vi "AlGaInPAs_Layer.vi"(2 "Debug Mode":bool, 3 "Elapsed Time (s)":dbl, 4 "State":enum16{"Edit", "Start", "Run", "End", "Idle"}(ring), 5 "Argument List In":string[](array[string])) -> (0 "Status Out":string, 1 "Argument List Out":string[](array[string]))   [LabVIEW 2011]
panel:
  out "Al?":bool
  out "In?":bool
  out "Ga?":bool
  out "AsH3?":bool
  out "PH3?":bool
  in  "AsH3 Flow":dbl
  in  "AsH3 run":bool
  in  "Al_run":bool
  in  "Al Flow":dbl
  in  "PH3 run":bool
  in  "In run":bool
  in  "Ga run":bool
  in  "PH3 Flow":dbl
  in  "In Flow":dbl
  in  "Ga Flow":dbl
  in  "Cancel":bool
  in  "OK":bool
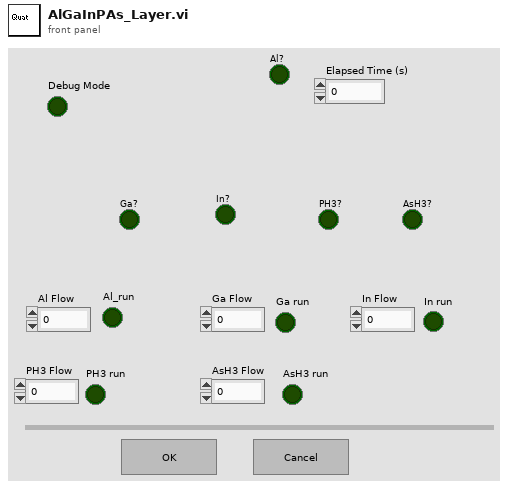
[diagram p1: front panel]
types:
  T1 = enum16{"Discrete", "Continuous", "Instantaneous"}
  T2 = enum32{"Invalid", "Default", "Floating", "Floating/Auto-Hide", "Modal"}
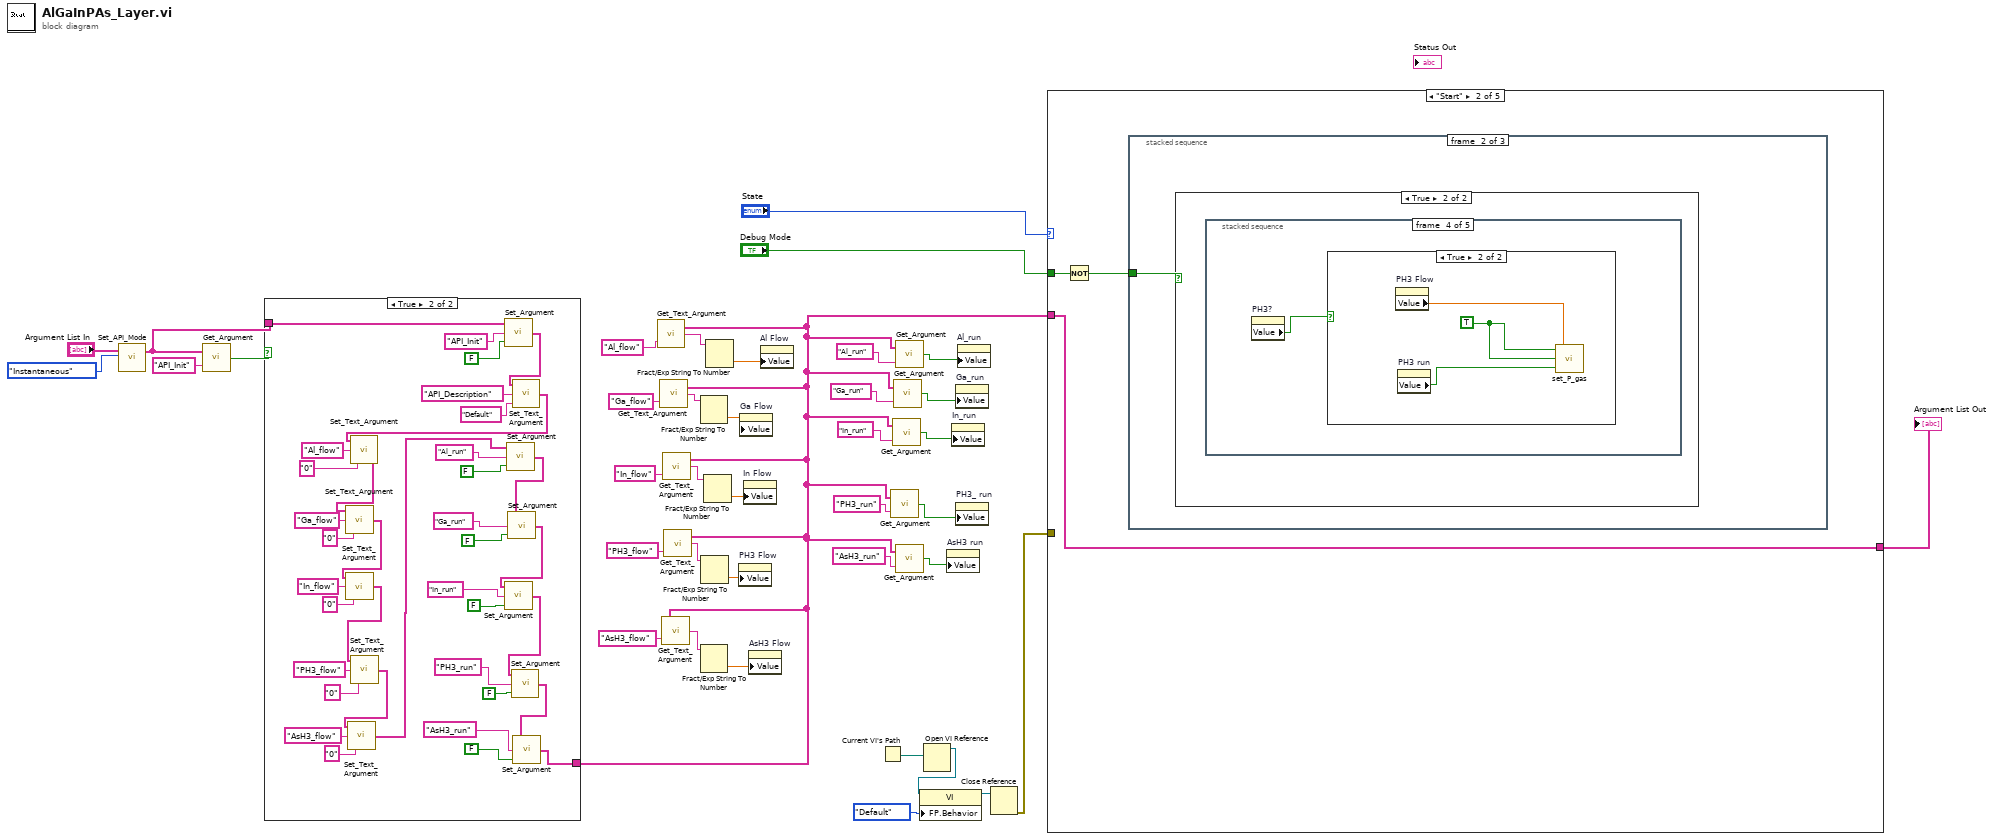
[diagram p0: block diagram]
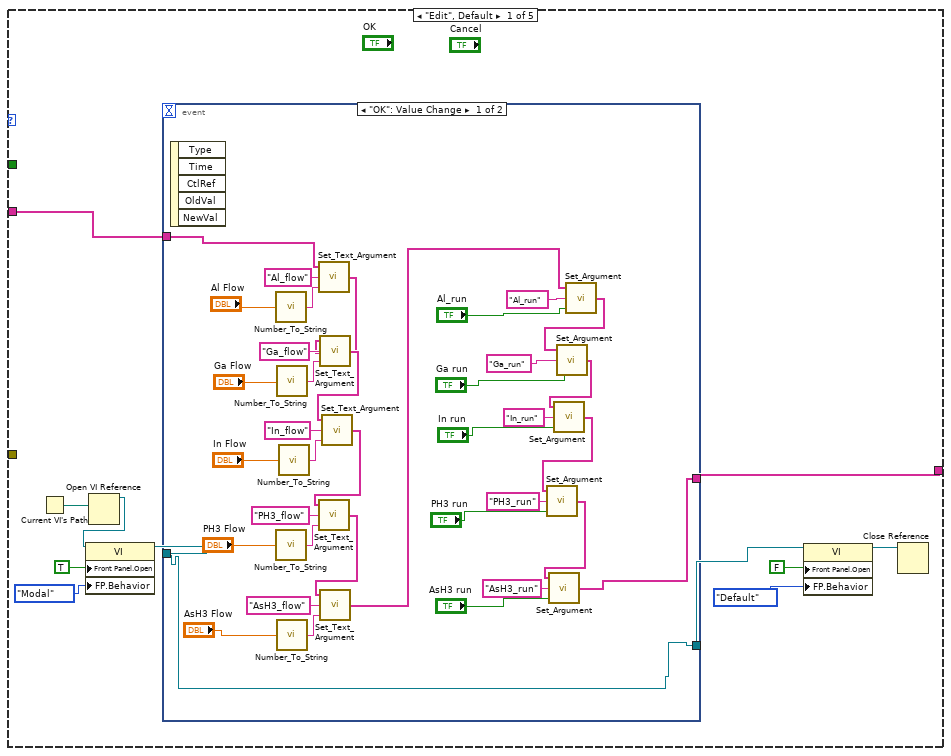
[diagram p3: hidden frame]
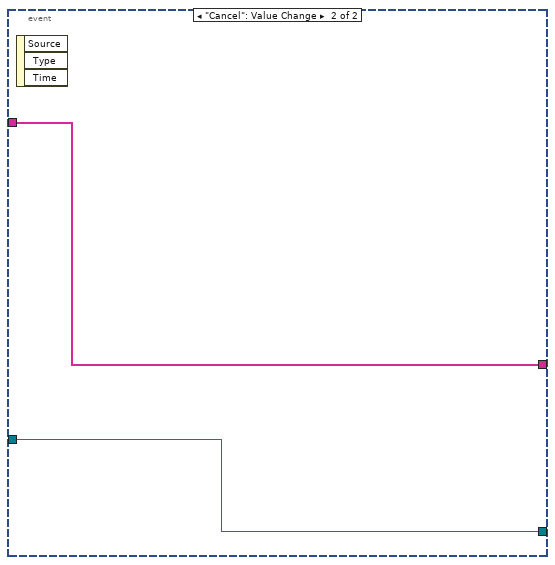
[diagram p4: hidden frame]
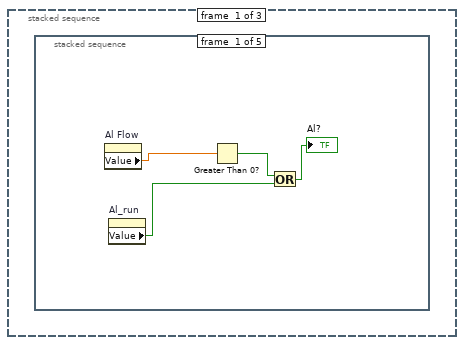
[diagram p5: hidden frame]
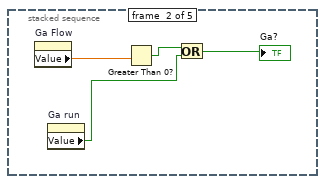
[diagram p6: hidden frame]
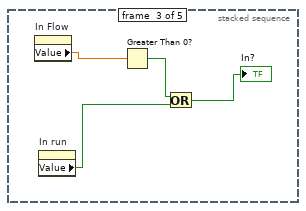
[diagram p7: hidden frame]
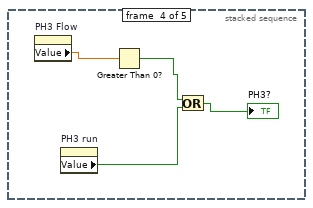
[diagram p8: hidden frame]
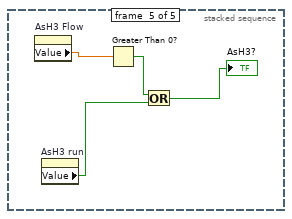
[diagram p9: hidden frame]
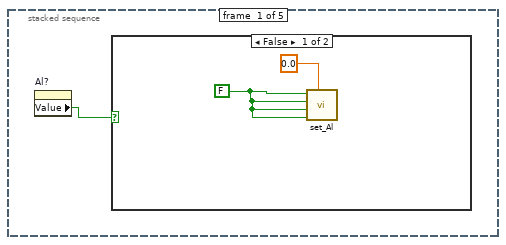
[diagram p11: hidden frame]
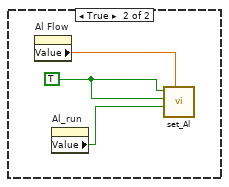
[diagram p12: hidden frame]
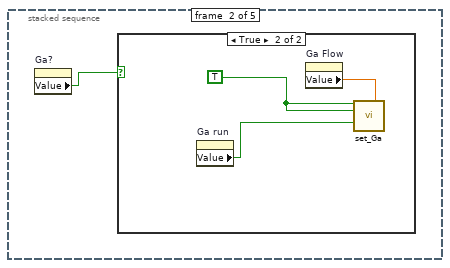
[diagram p13: hidden frame]
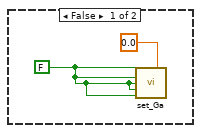
[diagram p14: hidden frame]
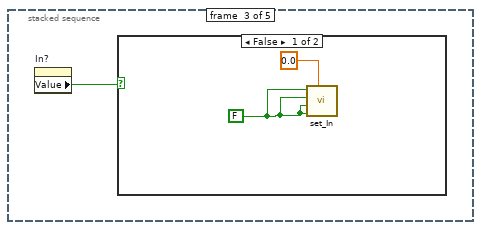
[diagram p15: hidden frame]
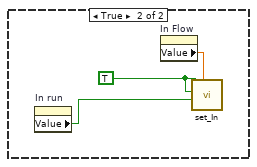
[diagram p16: hidden frame]
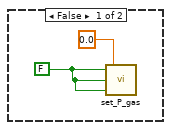
[diagram p17: hidden frame]
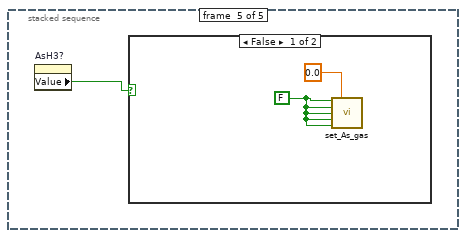
[diagram p18: hidden frame]
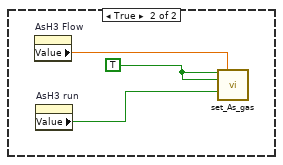
[diagram p19: hidden frame]
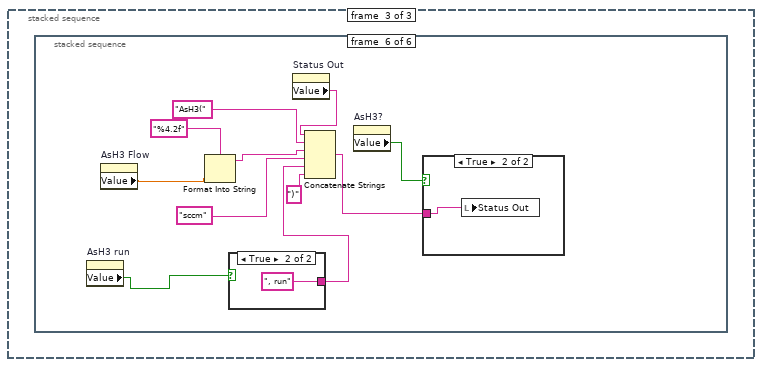
[diagram p20: hidden frame]
diagram:
  n1 = call "Set_API_Mode.vi"("API Mode"=T1."Instantaneous", "Argument List In"="Argument List In") -> ("Argument List Out"=w26:string[])  [unwired: 3 in]
  n2 = call "Get_Argument.vi"("Argument"="API_Init", "Argument List"=w26) -> ("Enabled"=w27:bool)
  n3 = case shown="True" w27 {
    tunnel: w26 -> [w40 w77]
    tunnel: [w40 w53] -> w1
    frame False {
    }
    frame True {
      n4 = call "Set_Argument.vi"("Enable"=FALSE, "Argument"="API_Init", "Argument List In"=w77) -> ("Argument List Out"=w74:string[])
      n5 = call "Set_Text_Argument.vi"("Text"="Default", "Argument"="API_Description", "Argument List In"=w74) -> ("Argument List Out"=w45:string[])
      n6 = call "Set_Text_Argument.vi"("Text"="0", "Argument"="Al_flow", "Argument List In"=w45) -> ("Argument List Out"=w44:string[])
      n7 = call "Set_Text_Argument.vi"("Text"="0", "Argument"="Ga_flow", "Argument List In"=w44) -> ("Argument List Out"=w67:string[])
      n8 = call "Set_Text_Argument.vi"("Text"="0", "Argument"="In_flow", "Argument List In"=w67) -> ("Argument List Out"=w43:string[])
      n9 = call "Set_Text_Argument.vi"("Text"="0", "Argument"="PH3_flow", "Argument List In"=w43) -> ("Argument List Out"=w55:string[])
      n10 = call "Set_Text_Argument.vi"("Text"="0", "Argument"="AsH3_flow", "Argument List In"=w55) -> ("Argument List Out"=w42:string[])
      n11 = call "Set_Argument.vi"("Enable"=FALSE, "Argument"="Al_run", "Argument List In"=w42) -> ("Argument List Out"=w48:string[])
      n12 = call "Set_Argument.vi"("Enable"=FALSE, "Argument"="Ga_run", "Argument List In"=w48) -> ("Argument List Out"=w58:string[])
      n13 = call "Set_Argument.vi"("Enable"=FALSE, "Argument"="In_run", "Argument List In"=w58) -> ("Argument List Out"=w41:string[])
      n14 = call "Set_Argument.vi"("Enable"=FALSE, "Argument"="PH3_run", "Argument List In"=w41) -> ("Argument List Out"=w51:string[])
      n15 = call "Set_Argument.vi"("Enable"=FALSE, "Argument"="AsH3_run", "Argument List In"=w51) -> ("Argument List Out"=w53:string[])
    }
  }
  n16 = call "Get_Text_Argument.vi"("Argument"="Al_flow", "Argument List"=w1) -> ("Text"=w6:string)
  n17 = call "Get_Text_Argument.vi"("Argument"="Ga_flow", "Argument List"=w1) -> ("Text"=w22:string)
  n18 = call "Get_Text_Argument.vi"("Argument"="AsH3_flow", "Argument List"=w1) -> ("Text"=w18:string)
  n19 = call "Get_Text_Argument.vi"("Argument"="In_flow", "Argument List"=w1) -> ("Text"=w20:string)
  n20 = call "Get_Text_Argument.vi"("Argument"="PH3_flow", "Argument List"=w1) -> ("Text"=w17:string)
  n21 = Fract/Exp String To Number(string=w22) -> (number=w21:dbl)  [unwired: 4 out]
  n22 = Fract/Exp String To Number(string=w18) -> (number=w2:dbl)  [unwired: 4 out]
  n23 = Fract/Exp String To Number(string=w17) -> (number=w16:dbl)  [unwired: 4 out]
  n24 = Fract/Exp String To Number(string=w20) -> (number=w19:dbl)  [unwired: 4 out]
  n25 = Fract/Exp String To Number(string=w6) -> (number=w3:dbl)  [unwired: 4 out]
  n26 = property on="PH3 Flow" class="DigNum (strict)"("Value"=w16) -> ()  [unwired: 2 in, 2 out]
  n27 = property on="Ga Flow" class="DigNum (strict)"("Value"=w21) -> ()  [unwired: 2 in, 2 out]
  n28 = property on="In Flow" class="DigNum (strict)"("Value"=w19) -> ()  [unwired: 2 in, 2 out]
  n29 = property on="AsH3 Flow" class="DigNum (strict)"("Value"=w2) -> ()  [unwired: 2 in, 2 out]
  n30 = property on="Al Flow" class="DigNum (strict)"("Value"=w3) -> ()  [unwired: 2 in, 2 out]
  n31 = Current VI's Path() -> (path=w35:path)
  n32 = call "Get_Argument.vi"("Argument"="PH3_run", "Argument List"=w1) -> ("Enabled"=w12:bool)
  n33 = call "Get_Argument.vi"("Argument"="In_run", "Argument List"=w1) -> ("Enabled"=w13:bool)
  n34 = call "Get_Argument.vi"("Argument"="Ga_run", "Argument List"=w1) -> ("Enabled"=w14:bool)
  n35 = call "Get_Argument.vi"("Argument"="Al_run", "Argument List"=w1) -> ("Enabled"=w5:bool)
  n36 = call "Get_Argument.vi"("Argument"="AsH3_run", "Argument List"=w1) -> ("Enabled"=w4:bool)
  n37 = Open VI Reference(vi path=w35) -> (vi reference=w34:refnum<vi>)  [unwired: 1 in, 5 out]
  n38 = property class="VI"(reference=w34, "FP.Behavior"=T2."Default" ("Front Panel Window:Behavior")) -> (reference out=w32:refnum<vi>)  [unwired: 1 in, 1 out]
  n39 = property on="AsH3 run" class="Bool (strict)"("Value"=w4) -> ()  [unwired: 2 in, 2 out]
  n40 = property on="In_run" class="Bool (strict)"("Value"=w13) -> ()  [unwired: 2 in, 2 out]
  n41 = property on="Ga_run" class="Bool (strict)"("Value"=w14) -> ()  [unwired: 2 in, 2 out]
  n42 = property on="PH3_ run" class="Bool (strict)"("Value"=w12) -> ()  [unwired: 2 in, 2 out]
  n43 = property on="Al_run" class="Bool (strict)"("Value"=w5) -> ()  [unwired: 2 in, 2 out]
  n44 = Close Reference(reference=w32) -> (error out=w31:errorcluster)  [unwired: 1 in]
  n45 = case shown="\"Start\"" "State" {
    tunnel: [w88 w130 w252 w253 w254] -> w38
    tunnel: w1 -> [w87 w130 w252 w253 w254]
    tunnel: "Debug Mode" -> [_ w129 _ _ _]
    tunnel: w31 -> [_ _ _ _ _]
    frame "Edit", Default {
      n46 = Current VI's Path() -> (path=w82:path)
      n47 = Open VI Reference(vi path=w82) -> (vi reference=w81:refnum<vi>)  [unwired: 1 in, 5 out]
      n48 = property class="VI"(reference=w81, "Front Panel.Open"=TRUE ("Front Panel Window:Open"), "FP.Behavior"=T2."Modal" ("Front Panel Window:Behavior")) -> (reference out=w85:refnum<vi>)  [unwired: 1 in, 1 out]
      n49 = event shown="[0] \"OK\": Value Change" {
        selector: _ -> [_ _]
        dyn-events: _ -> [_ _]
        timeout: _ -> [_ _]
        tunnel: w87 -> [w98 w126]
        tunnel: [w105 w126] -> w88
        tunnel: [w89 w127] -> w84
        tunnel: w85 -> [w89 w127]
        event "OK": Value Change {
          n50 = event-data() -> ()  [unwired: 6 out]
          n51 = call "Number_To_String.vi"("Number"="Al Flow") -> ("String"=w99:string)
          n52 = call "Number_To_String.vi"("Number"="PH3 Flow") -> ("String"=w117:string)
          n53 = call "Number_To_String.vi"("Number"="Ga Flow") -> ("String"=w124:string)
          n54 = call "Number_To_String.vi"("Number"="AsH3 Flow") -> ("String"=w95:string)
          n55 = call "Number_To_String.vi"("Number"="In Flow") -> ("String"=w121:string)
          n56 = call "Set_Text_Argument.vi"("Text"=w99, "Argument"="Al_flow", "Argument List In"=w98) -> ("Argument List Out"=w97:string[])
          n57 = call "Set_Text_Argument.vi"("Text"=w124, "Argument"="Ga_flow", "Argument List In"=w97) -> ("Argument List Out"=w120:string[])
          n58 = call "Set_Text_Argument.vi"("Text"=w121, "Argument"="In_flow", "Argument List In"=w120) -> ("Argument List Out"=w92:string[])
          n59 = call "Set_Text_Argument.vi"("Text"=w117, "Argument"="PH3_flow", "Argument List In"=w92) -> ("Argument List Out"=w93:string[])
          n60 = call "Set_Text_Argument.vi"("Text"=w95, "Argument"="AsH3_flow", "Argument List In"=w93) -> ("Argument List Out"=w94:string[])
          n61 = call "Set_Argument.vi"("Enable"="Al_run", "Argument"="Al_run", "Argument List In"=w94) -> ("Argument List Out"=w91:string[])
          n62 = call "Set_Argument.vi"("Enable"="Ga run", "Argument"="Ga_run", "Argument List In"=w91) -> ("Argument List Out"=w109:string[])
          n63 = call "Set_Argument.vi"("Enable"="In run", "Argument"="In_run", "Argument List In"=w109) -> ("Argument List Out"=w103:string[])
          n64 = call "Set_Argument.vi"("Enable"="PH3 run", "Argument"="PH3_run", "Argument List In"=w103) -> ("Argument List Out"=w104:string[])
          n65 = call "Set_Argument.vi"("Enable"="AsH3 run", "Argument"="AsH3_run", "Argument List In"=w104) -> ("Argument List Out"=w105:string[])
        }
        event "Cancel": Value Change {
          n66 = event-data() -> ()  [unwired: 4 out]
        }
      }
      n67 = property class="VI"(reference=w84, "Front Panel.Open"=FALSE ("Front Panel Window:Open"), "FP.Behavior"=T2."Default" ("Front Panel Window:Behavior")) -> (reference out=w78:refnum<vi>)  [unwired: 1 in, 1 out]
      n68 = Close Reference(reference=w78) -> ()  [unwired: 1 in, 1 out]
    }
    frame "Start" {
      n69 = Not(x=w129) -> (.not. x?=w128:bool)
      n70 = stacked-sequence {
        tunnel: w128 -> [_ w151 _]
        frame #0 {
          n71 = stacked-sequence {
            frame #0 {
              n72 = property on="Al Flow" class="DigNum (strict)"() -> ("Value"=w131:dbl)  [unwired: 2 in, 2 out]
              n73 = property on="Al_run" class="Bool (strict)"() -> ("Value"=w132:bool)  [unwired: 2 in, 2 out]
              n74 = Greater Than 0?(x=w131) -> (x > 0?=w134:bool)
              n75 = Or(x=w134, y=w132) -> (x .or. y?=→"Al?":bool)
            }
            frame #1 {
              n76 = property on="Ga Flow" class="DigNum (strict)"() -> ("Value"=w138:dbl)  [unwired: 2 in, 2 out]
              n77 = property on="Ga run" class="Bool (strict)"() -> ("Value"=w136:bool)  [unwired: 2 in, 2 out]
              n78 = Greater Than 0?(x=w138) -> (x > 0?=w137:bool)
              n79 = Or(x=w137, y=w136) -> (x .or. y?=→"Ga?":bool)
            }
            frame #2 {
              n80 = property on="In Flow" class="DigNum (strict)"() -> ("Value"=w142:dbl)  [unwired: 2 in, 2 out]
              n81 = property on="In run" class="Bool (strict)"() -> ("Value"=w140:bool)  [unwired: 2 in, 2 out]
              n82 = Greater Than 0?(x=w142) -> (x > 0?=w141:bool)
              n83 = Or(x=w141, y=w140) -> (x .or. y?=→"In?":bool)
            }
            frame #3 {
              n84 = property on="PH3 Flow" class="DigNum (strict)"() -> ("Value"=w146:dbl)  [unwired: 2 in, 2 out]
              n85 = property on="PH3 run" class="Bool (strict)"() -> ("Value"=w144:bool)  [unwired: 2 in, 2 out]
              n86 = Greater Than 0?(x=w146) -> (x > 0?=w145:bool)
              n87 = Or(x=w145, y=w144) -> (x .or. y?=→"PH3?":bool)
            }
            frame #4 {
              n88 = property on="AsH3 Flow" class="DigNum (strict)"() -> ("Value"=w150:dbl)  [unwired: 2 in, 2 out]
              n89 = property on="AsH3 run" class="Bool (strict)"() -> ("Value"=w148:bool)  [unwired: 2 in, 2 out]
              n90 = Greater Than 0?(x=w150) -> (x > 0?=w149:bool)
              n91 = Or(x=w149, y=w148) -> (x .or. y?=→"AsH3?":bool)
            }
          }
        }
        frame #1 {
          n92 = case shown="True" w151 {
            frame False {
            }
            frame True {
              n93 = stacked-sequence {
                frame #0 {
                  n94 = property on="Al?" class="Bool (strict)"() -> ("Value"=w152:bool)  [unwired: 2 in, 2 out]
                  n95 = case shown="False" w152 {
                    frame False {
                      w153 = FALSE ("Al Active")
                      n96 = call "set_Al.vi"("ALMFC1"=0.0 ("Aluminum Flow"), "Remote"=w153, "Run"=w153, "Bubbler In"=w153, "Active"=w153) -> ()  [unwired: 5 out]
                    }
                    frame True {
                      w157 = TRUE ("Al Active")
                      n97 = property on="Al Flow" class="DigNum (strict)"() -> ("Value"=w155:dbl)  [unwired: 2 in, 2 out]
                      n98 = property on="Al_run" class="Bool (strict)"() -> ("Value"=w156:bool)  [unwired: 2 in, 2 out]
                      n99 = call "set_Al.vi"("ALMFC1"=w155, "Run"=w156, "Bubbler In"=w157, "Active"=w157) -> ()  [unwired: 1 in, 5 out]
                    }
                  }
                }
                frame #1 {
                  n100 = property on="Ga?" class="Bool (strict)"() -> ("Value"=w158:bool)  [unwired: 2 in, 2 out]
                  n101 = case shown="True" w158 {
                    frame False {
                      w159 = FALSE ("Ga Active")
                      n102 = call "set_Ga.vi"("Active"=w159, "GAMFC1"=0.0 ("Ga Flow 1"), "Bubbler In"=w159, "H2 Dilute"=w159, "Run"=w159, "Remote"=w159) -> ()  [unwired: 2 in, 8 out]
                    }
                    frame True {
                      w163 = TRUE ("Ga Active")
                      n103 = property on="Ga run" class="Bool (strict)"() -> ("Value"=w162:bool)  [unwired: 2 in, 2 out]
                      n104 = property on="Ga Flow" class="DigNum (strict)"() -> ("Value"=w161:dbl)  [unwired: 2 in, 2 out]
                      n105 = call "set_Ga.vi"("Active"=w163, "GAMFC1"=w161, "Bubbler In"=w163, "Run"=w162) -> ()  [unwired: 4 in, 8 out]
                    }
                  }
                }
                frame #2 {
                  n106 = property on="In?" class="Bool (strict)"() -> ("Value"=w164:bool)  [unwired: 2 in, 2 out]
                  n107 = case shown="False" w164 {
                    frame False {
                      w166 = FALSE ("In Remote")
                      n108 = call "set_In.vi"("INMFC1"=0.0 ("Indium Flow"), "Remote"=w166, "Run"=w166, "Bubbler In"=w166, "Active"=w166) -> ()  [unwired: 5 out]
                    }
                    frame True {
                      w169 = TRUE ("In Run")
                      n109 = property on="In run" class="Bool (strict)"() -> ("Value"=w167:bool)  [unwired: 2 in, 2 out]
                      n110 = property on="In Flow" class="DigNum (strict)"() -> ("Value"=w168:dbl)  [unwired: 2 in, 2 out]
                      n111 = call "set_In.vi"("INMFC1"=w168, "Run"=w167, "Bubbler In"=w169, "Active"=w169) -> ()  [unwired: 1 in, 5 out]
                    }
                  }
                }
                frame #3 {
                  n112 = property on="PH3?" class="Bool (strict)"() -> ("Value"=w170:bool)  [unwired: 2 in, 2 out]
                  n113 = case shown="True" w170 {
                    frame False {
                      w171 = FALSE ("P_Gas Active")
                      n114 = call "set_P_gas.vi"("Run"=w171, "Gas In"=w171, "Active"=w171, "P_Gas Remote"=w171, "H2 Flush"=w171, "P_Gas Flow"=0.0) -> ()
                    }
                    frame True {
                      w175 = TRUE ("P_Gas Active")
                      n115 = property on="PH3 Flow" class="DigNum (strict)"() -> ("Value"=w174:dbl)  [unwired: 2 in, 2 out]
                      n116 = property on="PH3 run" class="Bool (strict)"() -> ("Value"=w173:bool)  [unwired: 2 in, 2 out]
                      n117 = call "set_P_gas.vi"("Active"=w175, "P_Gas Remote"=w173, "H2 Flush"=w175, "P_Gas Flow"=w174) -> ()  [unwired: 2 in]
                    }
                  }
                }
                frame #4 {
                  n118 = property on="AsH3?" class="Bool (strict)"() -> ("Value"=w176:bool)  [unwired: 2 in, 2 out]
                  n119 = case shown="False" w176 {
                    frame False {
                      w177 = FALSE ("As_Gas Active")
                      n120 = call "set_As_gas.vi"("Active"=w177, "As_Gas Flow"=0.0, "Gas In"=w177, "H2 Flush"=w177, "Run"=w177, "Remote"=w177) -> ()  [unwired: 10 out]
                    }
                    frame True {
                      w181 = TRUE ("As_Gas Active")
                      n121 = property on="AsH3 Flow" class="DigNum (strict)"() -> ("Value"=w179:dbl)  [unwired: 2 in, 2 out]
                      n122 = property on="AsH3 run" class="Bool (strict)"() -> ("Value"=w180:bool)  [unwired: 2 in, 2 out]
                      n123 = call "set_As_gas.vi"("Active"=w181, "As_Gas Flow"=w179, "Gas In"=w181, "Run"=w180) -> ()  [unwired: 2 in, 10 out]
                    }
                  }
                }
              }
            }
          }
        }
        frame #2 {
          n124 = stacked-sequence {
            frame #0 {
              n125 = local write "Status Out"("" ("Status Out")) -> ()
            }
            frame #1 {
              n126 = property on="Al_run" class="Bool (strict)"() -> ("Value"=w190:bool)  [unwired: 2 in, 2 out]
              n127 = property on="Al Flow" class="DigNum (strict)"() -> ("Value"=w186:dbl)  [unwired: 2 in, 2 out]
              n128 = Format Into String(format string="%4.1f", w186) -> (resulting string=w185:string)  [unwired: 2 in, 1 out]
              n129 = case shown="True" w190 {
                tunnel: ["" ", run"] -> w189
                frame False {
                }
                frame True {
                }
              }
              n130 = Concatenate Strings("Al(" ("string"), w185, "sccm" ("string"), w189, ")" ("string")) -> (w187:string)
              n131 = property on="Al?" class="Bool (strict)"() -> ("Value"=w183:bool)  [unwired: 2 in, 2 out]
              n132 = case shown="True" w183 {
                tunnel: w187 -> [_ w193]
                frame False {
                }
                frame True {
                  n133 = local write "Status Out"(w193) -> ()
                }
              }
            }
            frame #2 {
              n134 = property on="Ga run" class="Bool (strict)"() -> ("Value"=w198:bool)  [unwired: 2 in, 2 out]
              n135 = property on="Ga Flow" class="DigNum (strict)"() -> ("Value"=w199:dbl)  [unwired: 2 in, 2 out]
              n136 = Format Into String(format string="%4.1f", w199) -> (resulting string=w201:string)  [unwired: 2 in, 1 out]
              n137 = case shown="True" w198 {
                tunnel: ["" ", run"] -> w204
                frame False {
                }
                frame True {
                }
              }
              n138 = property on="Status Out" class="Str"() -> ("Value"=w196:string)  [unwired: 2 in, 2 out]
              n139 = Concatenate Strings(w196, "Ga(" ("string"), w201, "sccm" ("string"), w204, ")" ("string")) -> (w202:string)
              n140 = property on="Ga?" class="Bool (strict)"() -> ("Value"=w197:bool)  [unwired: 2 in, 2 out]
              n141 = case shown="True" w197 {
                tunnel: w202 -> [_ w207]
                frame False {
                }
                frame True {
                  n142 = local write "Status Out"(w207) -> ()
                }
              }
            }
            frame #3 {
              n143 = property on="In run" class="Bool (strict)"() -> ("Value"=w212:bool)  [unwired: 2 in, 2 out]
              n144 = property on="In Flow" class="DigNum (strict)"() -> ("Value"=w213:dbl)  [unwired: 2 in, 2 out]
              n145 = Format Into String(format string="%4.1f", w213) -> (resulting string=w215:string)  [unwired: 2 in, 1 out]
              n146 = property on="Status Out" class="Str"() -> ("Value"=w210:string)  [unwired: 2 in, 2 out]
              n147 = case shown="False" w212 {
                tunnel: ["" ", run"] -> w218
                frame False {
                }
                frame True {
                }
              }
              n148 = Concatenate Strings(w210, "In(" ("string"), w215, "sccm" ("string"), w218, ")" ("string")) -> (w216:string)
              n149 = property on="In?" class="Bool (strict)"() -> ("Value"=w211:bool)  [unwired: 2 in, 2 out]
              n150 = case shown="True" w211 {
                tunnel: w216 -> [_ w221]
                frame False {
                }
                frame True {
                  n151 = local write "Status Out"(w221) -> ()
                }
              }
            }
            frame #4 {
              n152 = property on="PH3 run" class="Bool (strict)"() -> ("Value"=w227:bool)  [unwired: 2 in, 2 out]
              n153 = property on="PH3 Flow" class="DigNum (strict)"() -> ("Value"=w228:dbl)  [unwired: 2 in, 2 out]
              n154 = Format Into String(format string="%4.1f", w228) -> (resulting string=w230:string)  [unwired: 2 in, 1 out]
              n155 = case shown="False" w227 {
                tunnel: ["" ", run"] -> w232
                frame False {
                }
                frame True {
                }
              }
              n156 = property on="Status Out" class="Str"() -> ("Value"=w225:string)  [unwired: 2 in, 2 out]
              n157 = Concatenate Strings(w225, "PH3(" ("string"), w230, "sccm" ("string"), w232, ")" ("string")) -> (w226:string)
              n158 = property on="PH3?" class="Bool (strict)"() -> ("Value"=w229:bool)  [unwired: 2 in, 2 out]
              n159 = case shown="True" w229 {
                tunnel: w226 -> [_ w235]
                frame False {
                }
                frame True {
                  n160 = local write "Status Out"(w235) -> ()
                }
              }
            }
            frame #5 {
              n161 = property on="AsH3 run" class="Bool (strict)"() -> ("Value"=w241:bool)  [unwired: 2 in, 2 out]
              n162 = property on="AsH3 Flow" class="DigNum (strict)"() -> ("Value"=w242:dbl)  [unwired: 2 in, 2 out]
              n163 = Format Into String(format string="%4.2f", w242) -> (resulting string=w243:string)  [unwired: 2 in, 1 out]
              n164 = case shown="True" w241 {
                tunnel: ["" ", run"] -> w246
                frame False {
                }
                frame True {
                }
              }
              n165 = property on="Status Out" class="Str"() -> ("Value"=w239:string)  [unwired: 2 in, 2 out]
              n166 = Concatenate Strings(w239, "AsH3(" ("string"), w243, "sccm" ("string"), w246, ")" ("string")) -> (w244:string)
              n167 = property on="AsH3?" class="Bool (strict)"() -> ("Value"=w240:bool)  [unwired: 2 in, 2 out]
              n168 = case shown="True" w240 {
                tunnel: w244 -> [_ w249]
                frame False {
                }
                frame True {
                  n169 = local write "Status Out"(w249) -> ()
                }
              }
            }
          }
        }
      }
    }
    frame "Run" {
    }
    frame "End" {
    }
    frame "Idle" {
    }
  }
  "Argument List Out" <- w38
